vi "XMLchannel.vi"(1 "HV Cluster":T2={"HV Power On/Off"=[FALSE, FALSE, FALSE, FALSE, FALSE, FALSE, FALSE, FALSE], "Set Voltage"=["0", "0", "0", "0", "0", "0", "0", "0"], "HV Tolerance (%)"=1.0, "Current"=[]}, 2 "Channel Cluster":T1={"det_type"=["", "", "", "", "", "", "", ""], "Serial numbers"=["", "", "", "", "", "", "", ""], "Sources"=["", "", "", "", "", "", "", ""], "Trigger level"=[4000, 4000, 4000, 4000, 4000, 4000, 4000, 4000], "Data Record On/Off"=[FALSE, FALSE, FALSE, FALSE, FALSE, FALSE, FALSE, FALSE, FALSE, FALSE, FALSE, FALSE, FALSE, FALSE, FALSE, FALSE], "Number of Channels"=8}, 3 "Previous XML string":string) -> (0 "Output String":string)   [LabVIEW 2012]
uses:
  hv cluster control.ctl
panel:
  out "Numeric":i32
  in  "Trigger level":i16[](array[numeric])=[4000, 4000, 4000, 4000, 4000, 4000, 4000, 4000] caption="Trigger"
  out "Channel On/Off":bool[](array[boolean])
  # "Channel 0"
  # "Channel 1"
  # "Channel 2"
  # "Channel 3"
  # "Channel 4"
  # "Channel 5"
  # "Channel 6"
  # "Channel 7"
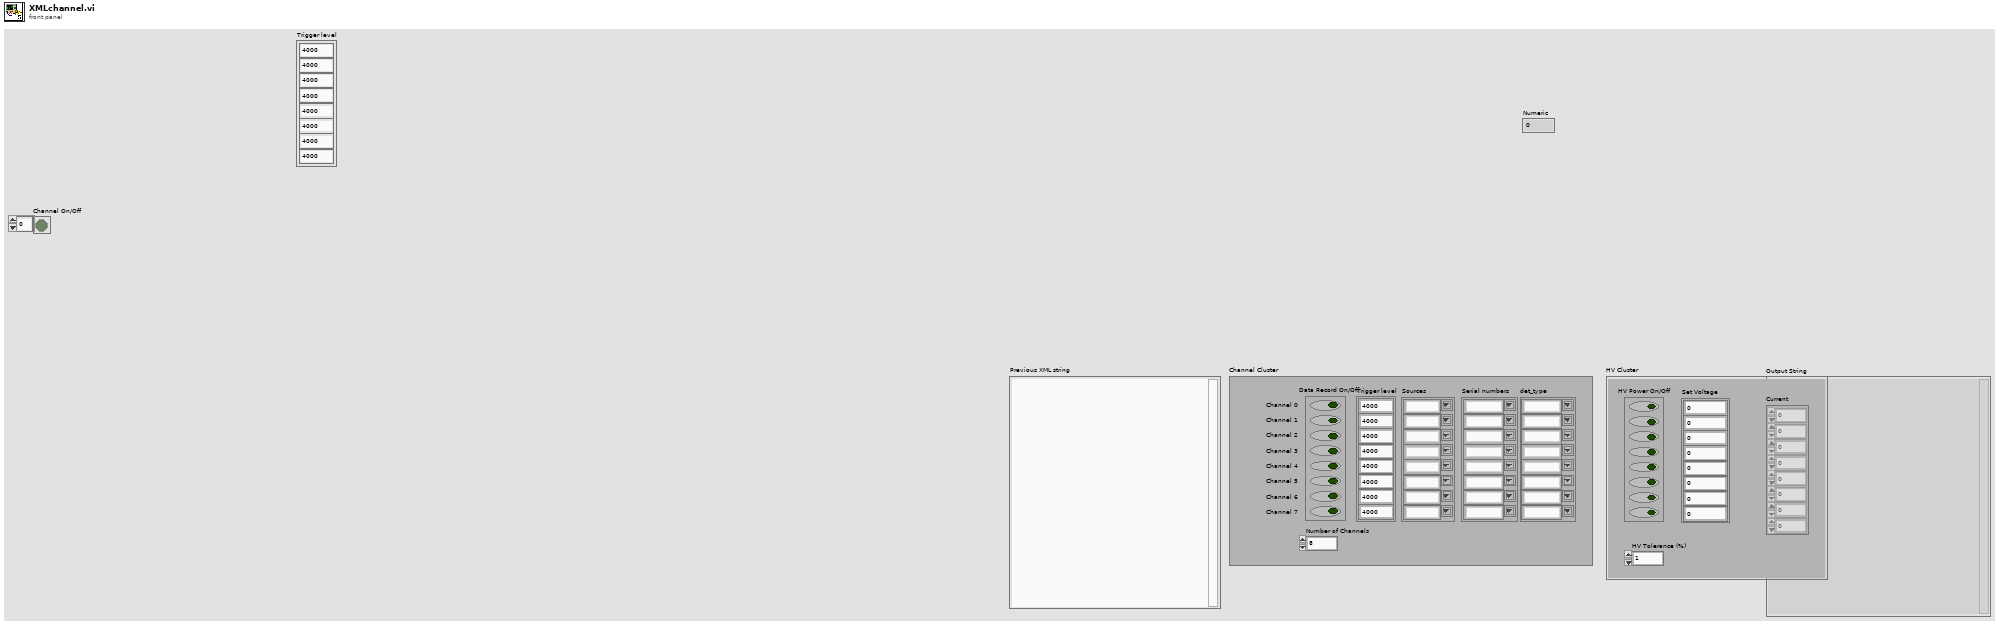
[diagram p1: front panel]
types:
  T1 = cluster{"det_type":string[], "Serial numbers":string[], "Sources":string[], "Trigger level":i16[], "Data Record On/Off":bool[], "Number of Channels":u8}
  T2 = typedef "hv cluster control.ctl" = cluster{"HV Power On/Off":bool[], "Set Voltage":string[], "HV Tolerance (%)":dbl, "Current":dbl[]}
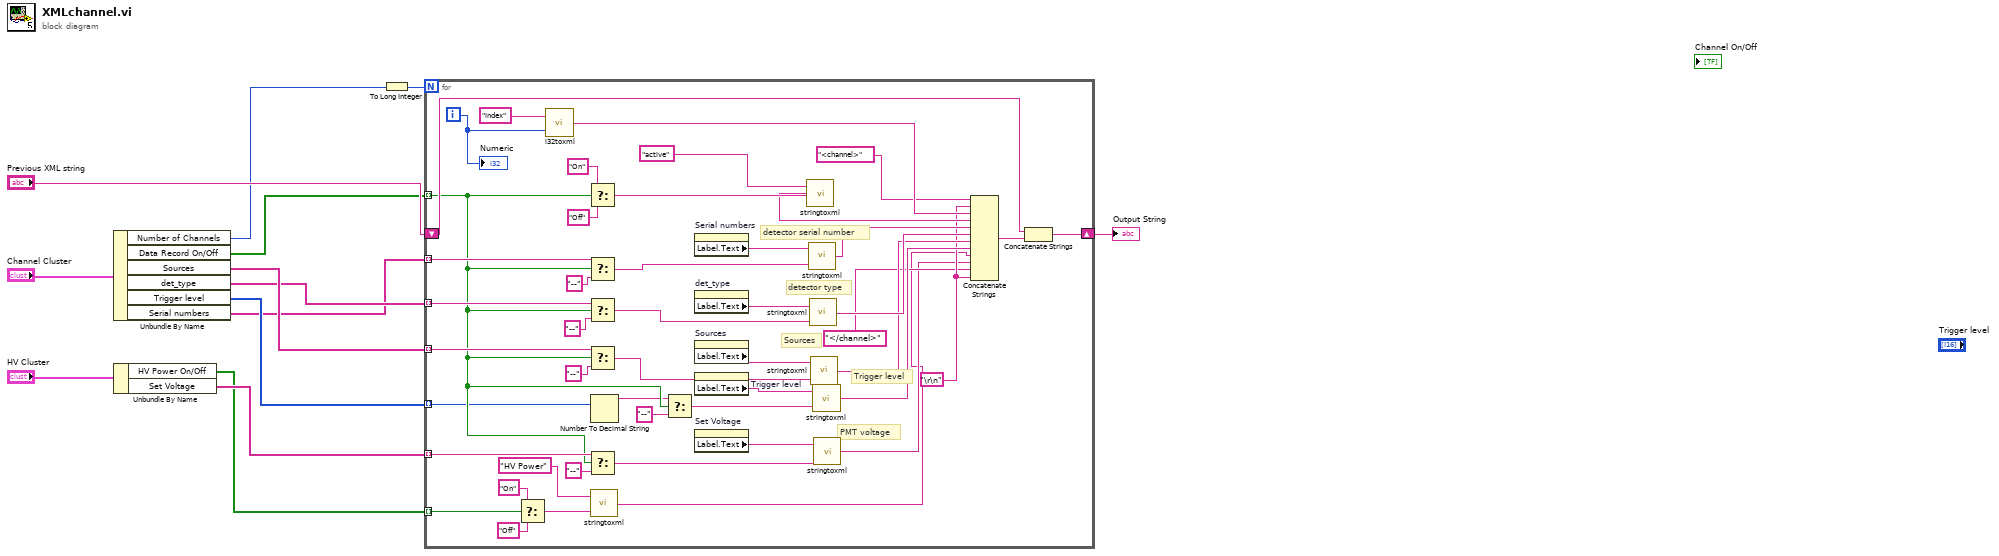
[diagram p0: block diagram]
diagram:
  n1 = Unbundle By Name("Channel Cluster") -> ("Number of Channels"=w3:u8, "Data Record On/Off"=w4:bool[], "Sources"=w12:string[], "det_type"=w11:string[], "Trigger level"=w10:i16[], "Serial numbers"=w8:string[])
  n2 = Unbundle By Name("HV Cluster") -> ("HV Power On/Off"=w6:bool[], "Set Voltage"=w7:string[])
  n3 = To Long Integer(number=w3) -> (32bit integer=w2:i32)
  n4 = for {
    N: w2 -> [_]
    shift-right: [w37] -> w9
    shift-left: "Previous XML string" -> [w36]
    tunnel: w4 -> [w30] mode=indexing
    tunnel: w12 -> [w33] mode=indexing
    tunnel: w11 -> [w34] mode=indexing
    tunnel: w8 -> [w32] mode=indexing
    tunnel: w10 -> [w29] mode=indexing
    tunnel: w7 -> [w31] mode=indexing
    tunnel: w6 -> [w27] mode=indexing
    i -> [w40]
    w22 = "\r\n"
    # "PMT voltage"
    # "Trigger level"
    # "Sources"
    # "detector type"
    # "detector serial number"
    n5 = Select(t="On" ("List Name"), s=w27, f="Off" ("List Name")) -> (s? t:f=w23:string)
    n6 = call "i32toxml.vi"("variable"=w40, "variable name"="index") -> ("xml string"=w55:string)
    n7 = Select(t="On" ("List Name"), s=w30, f="Off" ("List Name")) -> (s? t:f=w57:string)
    n8 = Select(t=w32, s=w30, f="--") -> (s? t:f=w52:string)
    n9 = Select(t=w34, s=w30, f="--") -> (s? t:f=w49:string)
    n10 = Select(t=w33, s=w30, f="--") -> (s? t:f=w46:string)
    n11 = Select(t=w31, s=w30, f="--") -> (s? t:f=w39:string)
    n12 = call "stringtoxml.vi"("String to write"=w23, "XML Tag"="HV Power") -> ("xml string"=w19:string)
    n13 = Number To Decimal String(number=w29) -> (decimal integer string=w28:string)  [unwired: 1 in]
    n14 = Select(t=w28, s=w30, f="--") -> (s? t:f=w43:string)
    n15 = property on="Serial numbers" class="Arr (strict)"() -> ("Label.Text"=w14:string)  [unwired: 2 in, 2 out]
    n16 = property on="det_type" class="Arr (strict)"() -> ("Label.Text"=w16:string)  [unwired: 2 in, 2 out]
    n17 = property on="Sources" class="Arr (strict)"() -> ("Label.Text"=w17:string)  [unwired: 2 in, 2 out]
    n18 = property on="Trigger level" class="Arr (strict)"() -> ("Label.Text"=w15:string)  [unwired: 2 in, 2 out]
    n19 = property on="Set Voltage" class="Arr (strict)"() -> ("Label.Text"=w18:string)  [unwired: 2 in, 2 out]
    n20 = call "stringtoxml.vi"("String to write"=w57, "XML Tag"="active") -> ("xml string"=w54:string)
    n21 = call "stringtoxml.vi"("String to write"=w52, "XML Tag"=w14) -> ("xml string"=w51:string)
    n22 = call "stringtoxml.vi"("String to write"=w49, "XML Tag"=w16) -> ("xml string"=w48:string)
    n23 = call "stringtoxml.vi"("String to write"=w46, "XML Tag"=w17) -> ("xml string"=w45:string)
    n24 = call "stringtoxml.vi"("String to write"=w43, "XML Tag"=w15) -> ("xml string"=w42:string)
    n25 = call "stringtoxml.vi"("String to write"=w39, "XML Tag"=w18) -> ("xml string"=w20:string)
    n26 = Concatenate Strings("<channel>" ("List Name"), w22, w55, w54, w51, w48, w45, w42, w19, w20, "</channel>" ("List Name"), w22) -> (w38:string)
    n27 = Concatenate Strings(w36, w38) -> (w37:string)
    "Numeric" <- w40
  }
  "Output String" <- w9
